vi "WriteGroup.vi"(11 "groupName":string) -> ()   [LabVIEW 2013]
doc: "WriteGroup assigns an array of given values to a group of tags."
uses:
  <vilib>/wsapi/Web Request.lvclass
  <vilib>/NI/TagWebClient/API/JSON Formats/ReadGroup Results.ctl
  <vilib>/NI/TagWebClient/API/JSON Formats/group type.ctl
  <vilib>/NI/TagWebClient/API/tagweb client API.lvlib
panel:
  in  "LabVIEW Web Service Request":refnum<class "Web Request.lvclass">
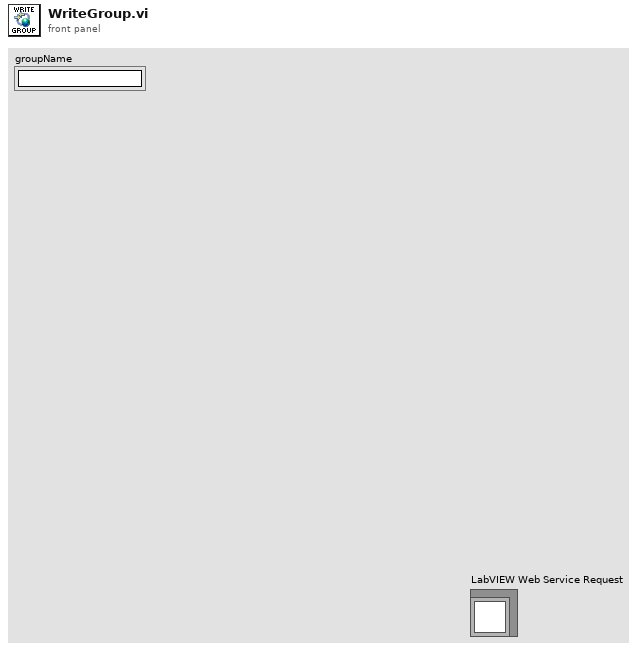
[diagram p1: front panel]
types:
  T1 = typedef "tagweb client API.lvlib/ReadGroup Results.ctl" = cluster{"data":T2[]}
  T2 = typedef "tagweb client API.lvlib/group type.ctl" = cluster{"type":string, "Values":string[]}
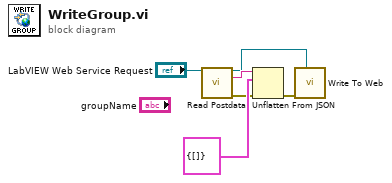
[diagram p0: block diagram]
diagram:
  n1 = call <vilib>:"Read Postdata.vi"("LabVIEW Web Service Request"="LabVIEW Web Service Request") -> ("LabVIEW Web Service Request out"=w1:refnum<class "Web Request.lvclass">, "postdata"=w6:string, "error out"=w3:errorcluster)  [unwired: 12 in]
  n2 = Unflatten From JSON(JSON string=w6, type and defaults=T1 {"data"=[]} ("Read Group Results"), error in (no error)=w3) -> (error out=w4:errorcluster)  [unwired: 4 in, 1 out]
  n3 = call <vilib>:"Write To Web.vi"("Web Request in"=w1, "error in"=w4) -> ()  [unwired: 10 in]
